vi "DAQ Channel Dlg_V0.vi"(7 "DAQ Sample Rate (S/s)":i32=100, 10 "Device Name":tag) -> (2 "Chl Infor":variant)   [LabVIEW 2021]
doc: "This vi helps to check if channels are in valid range and pass Channel Information out as a variant."
uses:
  Control/Volt Chl.ctl
panel:
  in  "OK Button":bool
  in  "Channel Array":T1(array[cluster])=[{"Ch"=0, "Desc"="Channel 0:", "Scale"=1.0, "Offset"=0.0, "Selected"=FALSE}, {"Ch"=1, "Desc"="Channel 1:", "Scale"=1.0, "Offset"=0.0, "Selected"=FALSE}, {"Ch"=2, "Desc"="Channel 2:", "Scale"=1.0, "Offset"=0.0, "Selected"=FALSE}, {"Ch"=3, "Desc"="Channel 3:", "Scale"=1.0, "Offset"=0.0, "Selected"=FALSE}, {"Ch"=4, "Desc"="Channel 4:", "Scale"=1.0, "Offset"=0.0, "Selected"=FALSE}, {"Ch"=5, "Desc"="Channel 5:", "Scale"=1.0, "Offset"=0.0, "Selected"=FALSE}, {"Ch"=6, "Desc"="Channel 6:", "Scale"=1.0, "Offset"=0.0, "Selected"=FALSE}, {"Ch"=7, "Desc"="Channel 7:", "Scale"=1.0, "Offset"=0.0, "Selected"=FALSE}, {"Ch"=8, "Desc"="", "Scale"=1.0, "Offset"=0.0, "Selected"=FALSE}, {"Ch"=9, "Desc"="", "Scale"=1.0, "Offset"=0.0, "Selected"=FALSE}, {"Ch"=10, "Desc"="", "Scale"=1.0, "Offset"=0.0, "Selected"=FALSE}, {"Ch"=11, "Desc"="", "Scale"=1.0, "Offset"=0.0, "Selected"=FALSE}, {"Ch"=12, "Desc"="", "Scale"=1.0, "Offset"=0.0, "Selected"=FALSE}, {"Ch"=13, "Desc"="", "Scale"=1.0, "Offset"=0.0, "Selected"=FALSE}, {"Ch"=14, "Desc"="", "Scale"=1.0, "Offset"=0.0, "Selected"=FALSE}, {"Ch"=15, "Desc"="", "Scale"=1.0, "Offset"=0.0, "Selected"=FALSE}]
  # "Ch"
  # "Description"
  # "Scale"
  # "Offset"
  # "Select Ch"
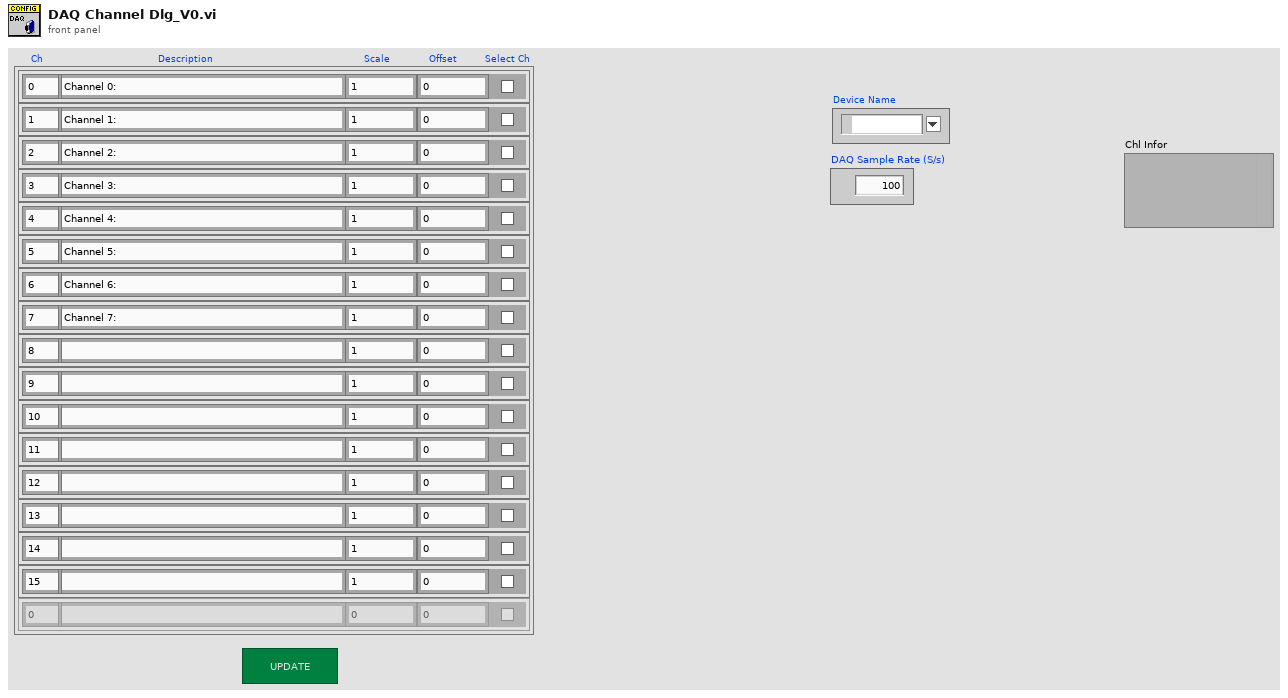
[diagram p1: front panel]
types:
  T1 = cluster{"Ch":i32, "Desc":string, "Scale":dbl, "Offset":dbl, "Selected":bool}[]
  T2 = typedef "Volt Chl.ctl" = cluster{"Index":i32[], "Chl Name":string[], "Scale":dbl[], "Offset":dbl[], "Sample Rate":i32, "Device Name":tag, "Channel":tag}
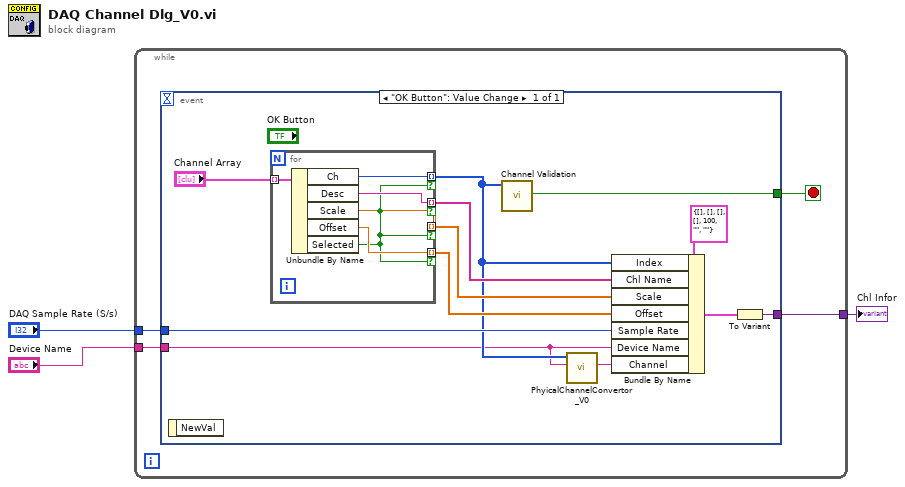
[diagram p0: block diagram]
diagram:
  n1 = while {
    tunnel: "DAQ Sample Rate (S/s)" -> [w6]
    tunnel: "Device Name" -> [w5]
    tunnel: [w4] -> w1
    stop <- w7 stop-if-true
    n2 = event shown="[0] \"OK Button\": Value Change" {
      selector: _ -> [_]
      dyn-events: _ -> [_]
      timeout: _ -> [_]
      tunnel: [w15] -> w7
      tunnel: w6 -> [w14]
      tunnel: w5 -> [w11]
      tunnel: [w9] -> w4
      event "OK Button": Value Change {
        n3 = event-data() -> ()  [unwired: 1 in, 1 out]
        n4 = for {
          tunnel: "Channel Array" -> [w25] mode=indexing
          tunnel: [w24] -> w13 mode=indexing if=w20
          tunnel: [w23] -> w18 mode=indexing if=w20
          tunnel: [w22] -> w17 mode=indexing if=w20
          tunnel: [w21] -> w16 mode=indexing if=w20
          n5 = Unbundle By Name(w25) -> ("Ch"=w24:i32, "Desc"=w23:string, "Scale"=w22:dbl, "Offset"=w21:dbl, "Selected"=w20:bool)
        }
        n6 = call "Channel Validation.vi"("User Defined Channels"=w13) -> ("Chl Valid?"=w15:bool)  [unwired: 10 in]
        n7 = call "PhyicalChannelConvertor_V0.vi"("Device Name"=w11, "Channel Number Array"=w13) -> ("physical channels"=w12:tag)  [unwired: 9 in]
        n8 = Bundle By Name(cluster=T2 {"Index"=[], "Chl Name"=[], "Scale"=[], "Offset"=[], "Sample Rate"=100, "Device Name"="", "Channel"=""}, "Index"=w13, "Chl Name"=w18, "Scale"=w17, "Offset"=w16, "Sample Rate"=w14, "Device Name"=w11, "Channel"=w12) -> (w10:T2)
        n9 = To Variant(anything=w10) -> (Variant=w9:variant)
      }
    }
  }
  "Chl Infor" <- w1
